vi "Install Octave Package golpi.vi"(6 "Verbose? (T)":bool=TRUE, 7 "Feature name":string="Bitstream data transfer mode", 8 "error in":errorcluster, 11 "GOLPI ref. in":T1={"pipe handle"={"lv_proc.dll file path"=path "", "process instance handle"=[], "debug mode"=FALSE, "debug data"=[]}, "fast read timeout [ms]"=500, "fast read settle time [ms]"=10, "fast read to multiple [ms]"=1, "max elements per input line"=100, "slow read timeout [ms]"=5000, "stdin double format specifier"="", "max elements per stdout output column"=100, "console mode bitstream"=FALSE, "bitstream first read timeout [ms]"=1000, "bitstream read timeout [ms]"=50, "struct transfer possible"=FALSE}) -> (0 "error out":errorcluster, 3 "GOLPI ref. out":T1={"pipe handle"={"lv_proc.dll file path"=path "", "process instance handle"=[], "debug mode"=FALSE, "debug data"=[]}, "fast read timeout [ms]"=500, "fast read settle time [ms]"=10, "fast read to multiple [ms]"=1, "max elements per input line"=100, "slow read timeout [ms]"=5000, "stdin double format specifier"="", "max elements per stdout output column"=100, "console mode bitstream"=FALSE, "bitstream first read timeout [ms]"=1000, "bitstream read timeout [ms]"=50, "struct transfer possible"=FALSE})   [LabVIEW 2013, in "GOLPI library.lvlib"]
doc: "Install GNU Octave package golpi. This package is required for Bitstream data transfer mode and for transfer of GNU Octave structures to LabVIEW clusters. VI search for package file golpi-X.X.X.tar.gz in application directory and subdirectories. If not found, a file dialog is opened for user to determine position of file. Input \"Feature name\" is used in description of message box. Input Verbose disables message box and file dialog.\n\n---\nGOLPI works only with lv_proc.dll library, which is part of vipm package or should be delivered together with packed library. Placement of this dll is selected in terminal of Start GNU Octave.vi."
uses:
  GOLPI library.lvlib
  Public/GOLPI reference Type Def.ctl
  LV Process source distribution/Pipe Handle.ctl
  Type Definitions/Custom Error Codes Enum Type Def.vi
  <vilib>/regexp/Match Regular Expression.xnode
  LV Process source distribution/LV Process library.lvlib
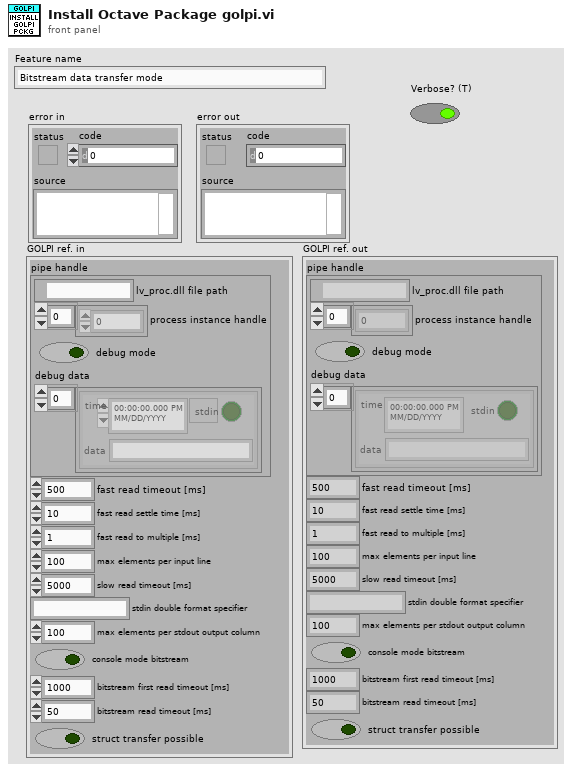
[diagram p1: front panel]
types:
  T1 = typedef "GOLPI library.lvlib/GOLPI reference Type Def.ctl" = cluster{"pipe handle":T2, "fast read timeout [ms]":u32, "fast read settle time [ms]":u32, "fast read to multiple [ms]":u32, "max elements per input line":u32, "slow read timeout [ms]":u32, "stdin double format specifier":string, "max elements per stdout output column":u32, "console mode bitstream":bool, "bitstream first read timeout [ms]":u32, "bitstream read timeout [ms]":u32, "struct transfer possible":bool}
  T2 = typedef "LV Process library.lvlib/Pipe Handle.ctl" = cluster{"lv_proc.dll file path":path, "process instance handle":u32[], "debug mode":bool, "debug data":cluster{"time":timestamp, "stdin":bool, "data":string}[]}
  T3 = typedef "GOLPI library.lvlib/Custom Error Codes Enum Type Def.vi" = enum16{"no error", "00 working directory PAR1 missing", "01 octave binary PAR1 missing", "02 octave report error PAR1", "03 empty output last cmd PAR1", "04 missing temporary file PAR1", "05 pwd PAR 1 not exist", "06 oct package not installed", "10 var PAR1 not string, vect", "11 var PAR1 not num, scal, ~compl", "12 var PAR1 not num, scal, compl", "13 var PAR1 not num, vect, ~compl", "14 var PAR1 not num, vect, compl", "15 var PAR1 not num, mat, ~compl", "16 var PAR1 not num, mat, ~compl", "30 read timeout", "60 bitstream transport failed", "61 bitstream decode error PAR1", "62 bitstream cannot be set", "70 struct transfer not possible", "80 struct: cluster elem. PAR1 not implem.", "81 struct: structure field PAR1 not implem.", "82 struct: size mismatch of PAR1", "83 struct: type mismatch of PAR1", "98 internal error", "99 not finished"}
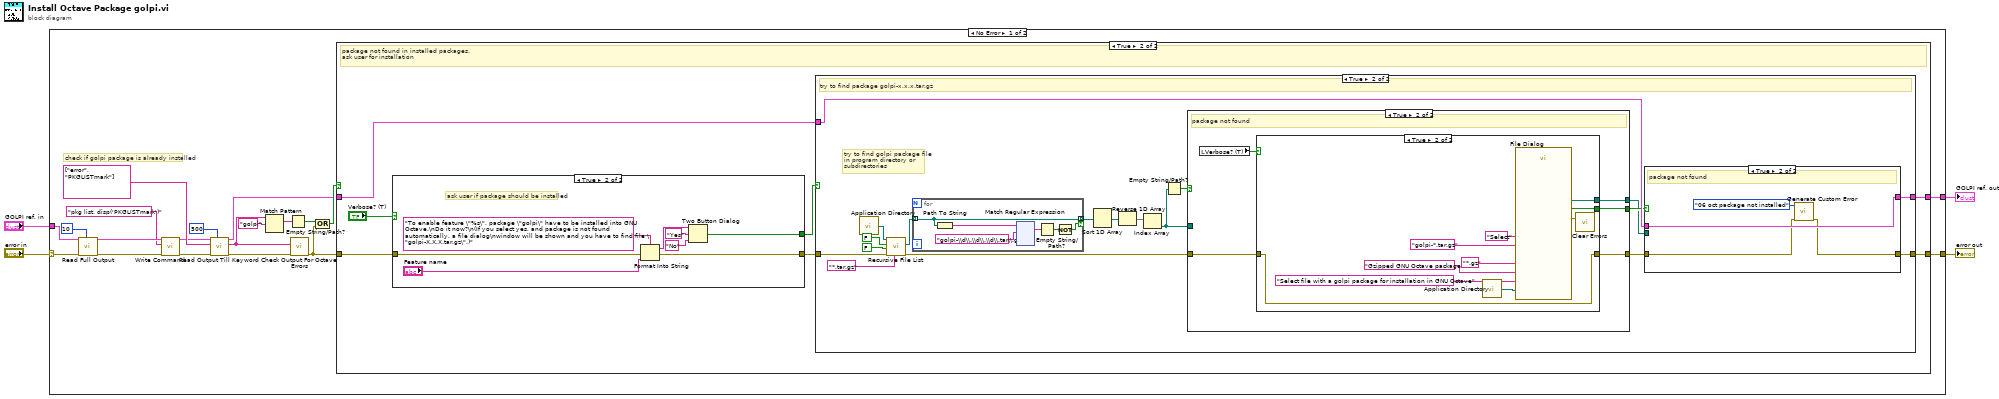
[diagram p0: block diagram]
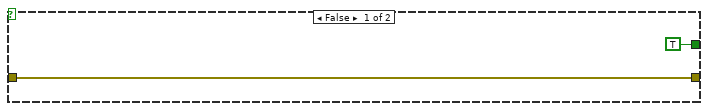
[diagram p3: hidden frame]
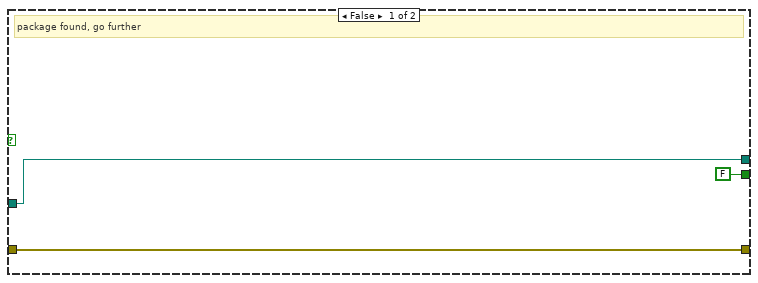
[diagram p5: hidden frame]
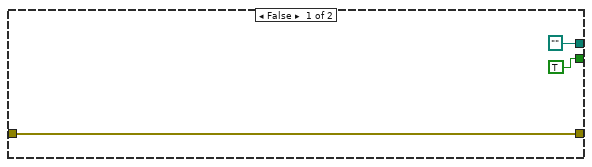
[diagram p6: hidden frame]
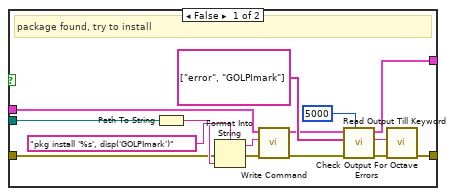
[diagram p7: hidden frame]
diagram:
  n1 = case shown="No Error" "error in" {
    selector: "error in" -> [w23 w225]
    tunnel: "GOLPI ref. in" -> [w24 w224]
    tunnel: [w9 w224] -> w3
    tunnel: [w22 w225] -> w1
    frame No Error {
      # "check if golpi package is already installed"
      n2 = call "Read Full Output.vi"("timeout [ms]"=u32 10, "error in"=w23, "GOLPI ref. in"=w24) -> ("error out"=w20:errorcluster, "GOLPI ref. out"=w21:T1)  [unwired: 5 in, 2 out]
      n3 = call "Write Command.vi"("error in"=w20, "command"="pkg list, disp('PKGLISTmark')", "GOLPI ref. in"=w21) -> ("error out"=w16:errorcluster, "GOLPI ref. out"=w15:T1)  [unwired: 7 in]
      n4 = call "Read Output Till Keyword.vi"("timeout [ms]"=u32 500, "error in"=w16, "keywords"=string[] ["error", "PKGLISTmark"], "GOLPI ref. in"=w15) -> ("error out"=w6:errorcluster, "read buffer"=w5:string, "GOLPI ref. out"=w10:T1)  [unwired: 4 in, 1 out]
      n5 = Match Pattern(string=w5, regular expression="golpi") -> (match substring=w7:string)  [unwired: 1 in, 3 out]
      n6 = Empty String/Path?(string/path=w7) -> (empty?=w17:bool)
      n7 = call "Check Output For Octave Errors.vi"("error in"=w6, "read buffer"=w5) -> ("error out"=w11:errorcluster)  [unwired: 9 in]
      n8 = Compound Arithmetic op=OR(w17, w11) -> (w13:bool)
      n9 = case shown="True" w13 {
        tunnel: [w26 w29] -> w22
        tunnel: w11 -> [w26 w33]
        tunnel: w10 -> [w25 w30]
        tunnel: [w25 w28] -> w9
        frame False {
          # "package seems to be already installed,\nnothing to do"
        }
        frame True {
          # "package not found in installed packages,\nask user for installation"
          n10 = case shown="True" "Verbose? (T)" {
            tunnel: w33 -> [w34 w40]
            tunnel: [TRUE ("T button?") w37] -> w32
            tunnel: [w34 w36] -> w31
            frame False {
            }
            frame True {
              # "ask user if package should be installed"
              n11 = Format Into String(format string="To enable feature \"%s\", package \"golpi\" have to be installed into GNU Octave.\nDo it now?\n(If you select yes, and package is not found automatically, a file dialog\nwindow will be shown and you have to find file \"golpi-X.X.X.tar.gz\".)" ("message"), error in=w40, "Feature name") -> (resulting string=w38:string, error out=w36:errorcluster)  [unwired: 1 in]
              n12 = Two Button Dialog(message=w38, 1:"No" ("F button name (\"Cancel\")"), 2:"Yes" ("T button name (\"OK\")")) -> (T button?=w37:bool)
            }
          }
          n13 = case shown="True" w32 {
            tunnel: w31 -> [w45 w50]
            tunnel: w30 -> [w44 w58]
            tunnel: [w45 w47] -> w29
            tunnel: [w44 w46] -> w28
            frame False {
              # "user do not want to install package, nothing to do, no error to generate."
            }
            frame True {
              # "try to find golpi package file\nin program directory or\nsubdirectories"
              # "try to find package golpi-x.x.x.tar.gz"
              n14 = call <vilib>:"Application Directory.vi"() -> ("Application Directory"=w63:path)
              n15 = call <vilib>:"Recursive File List.vi"("pattern"="*.tar.gz", "error in (no error)"=w50, "Continue Recursing on Error? (F)"=FALSE, "Treat LLBs as Folders?"=FALSE, "Folder Path"=w63) -> ("error out"=w49:errorcluster, "All Files in Dir"=w62:path[])  [unwired: 2 in, 3 out]
              n16 = for {
                tunnel: w62 -> [w106] mode=indexing
                tunnel: [w106] -> w61 mode=indexing if=w105
                n17 = Path To String(path=w106) -> (string=w104:string)
                n18 = xnode "Match Regular Expression"("input string"=w104, "regular expression"="golpi-\\d\\.\\d\\.\\d\\.tar\\.gz") -> ("whole match"=w108:string)  [unwired: 4 in, 4 out]
                n19 = Empty String/Path?(string/path=w108) -> (empty?=w107:bool)
                n20 = Not(x=w107) -> (.not. x?=w105:bool)
              }
              n21 = Sort 1D Array(array=w61) -> (sorted array=w60:path[])
              n22 = Reverse 1D Array(array=w60) -> (reversed array=w59:path[])
              n23 = Index Array(array=w59) -> (element=w55:path)  [unwired: 1 in]
              n24 = Empty String/Path?(string/path=w55) -> (empty?=w57:bool)
              n25 = case shown="True" w57 {
                tunnel: [FALSE w71] -> w56
                tunnel: [w65 w70] -> w54
                tunnel: w55 -> [w65 _]
                tunnel: w49 -> [w64 w69]
                tunnel: [w64 w68] -> w53
                frame False {
                  # "package found, go further"
                }
                frame True {
                  # "package not found"
                  n26 = local read "Verbose? (T)"() -> (w67:bool)
                  n27 = case shown="True" w67 {
                    tunnel: [TRUE ("cancelled") w78] -> w71
                    tunnel: [path "" w77] -> w70
                    tunnel: w69 -> [w74 w76]
                    tunnel: [w74 w76] -> w68
                    frame False {
                    }
                    frame True {
                      n28 = call <vilib>:"Application Directory.vi"() -> ("Application Directory"=w79:path)
                      n29 = call "File Dialog"("start path"=w79, "prompt"="Select file with a golpi package for installation in GNU Octave", "button label"="Select", "default name"="golpi-*.tar.gz", "pattern (all files)"="*.gz", "pattern label"="Gzipped GNU Octave package") -> ("selected path"=w77:path, "cancelled"=w78:bool, "error out"=w75:errorcluster)  [unwired: 6 in, 1 out]
                      n30 = call <vilib>:"Clear Errors.vi"("error in (no error)"=w75) -> ()  [unwired: 6 in, 1 out]
                    }
                  }
                }
              }
              n31 = case shown="True" w56 {
                tunnel: w53 -> [w88 w101]
                tunnel: w58 -> [w93 w103]
                tunnel: w54 -> [w92 _]
                tunnel: [w86 w100] -> w47
                tunnel: [w85 w103] -> w46
                frame False {
                  # "package found, try to install"
                  n32 = Path To String(path=w92) -> (string=w90:string)
                  n33 = Format Into String(format string="pkg install '%s', disp('GOLPImark')" ("command"), error in=w88, w90) -> (resulting string=w89:string, error out=w87:errorcluster)  [unwired: 1 in]
                  n34 = call "Write Command.vi"("error in"=w87, "command"=w89, "GOLPI ref. in"=w93) -> ("error out"=w98:errorcluster, "GOLPI ref. out"=w97:T1)  [unwired: 7 in]
                  n35 = call "Read Output Till Keyword.vi"("timeout [ms]"=u32 5000, "error in"=w98, "keywords"=string[] ["error", "GOLPImark"], "GOLPI ref. in"=w97) -> ("error out"=w95:errorcluster, "read buffer"=w94:string, "GOLPI ref. out"=w85:T1)  [unwired: 4 in, 1 out]
                  n36 = call "Check Output For Octave Errors.vi"("error in"=w95, "read buffer"=w94) -> ("error out"=w86:errorcluster)  [unwired: 9 in]
                }
                frame True {
                  # "package not found"
                  n37 = call "Generate Custom Error.vi"("error in"=w101, "GOLPI error"=Custom_Error_Codes_Enum_Type_Def.vi."06 oct package not installed") -> ("error out"=w100:errorcluster)  [unwired: 9 in]
                }
              }
            }
          }
        }
      }
    }
    frame Error {
    }
  }
  "error out" <- w1
  "GOLPI ref. out" <- w3
